vi "CoolProp_LogPH_SUBVI.vi"(9 "appended path":path, 10 "HoejTryk":dbl=-1111111111.0 format="%#.6f", 11 "Lavtryk":dbl=-1111111111.0 format="%#.6f") -> (0 "LogPH":cluster{dbl[], dbl[]}[](array[cluster]), 1 "Punkt4":T1, 2 "Punkt3":T1, 3 "Punkt1":T1, 5 "Punkt2":T1)   [LabVIEW 2022 SP3]
uses:
  Coolprop_64bit/CoolProp_advanced.llb/FluidCommon.ctl
  Coolprop_64bit/CoolProp_advanced.llb/FluidOfInterest.ctl
  Coolprop_64bit/Coolprop_lib.lvlib
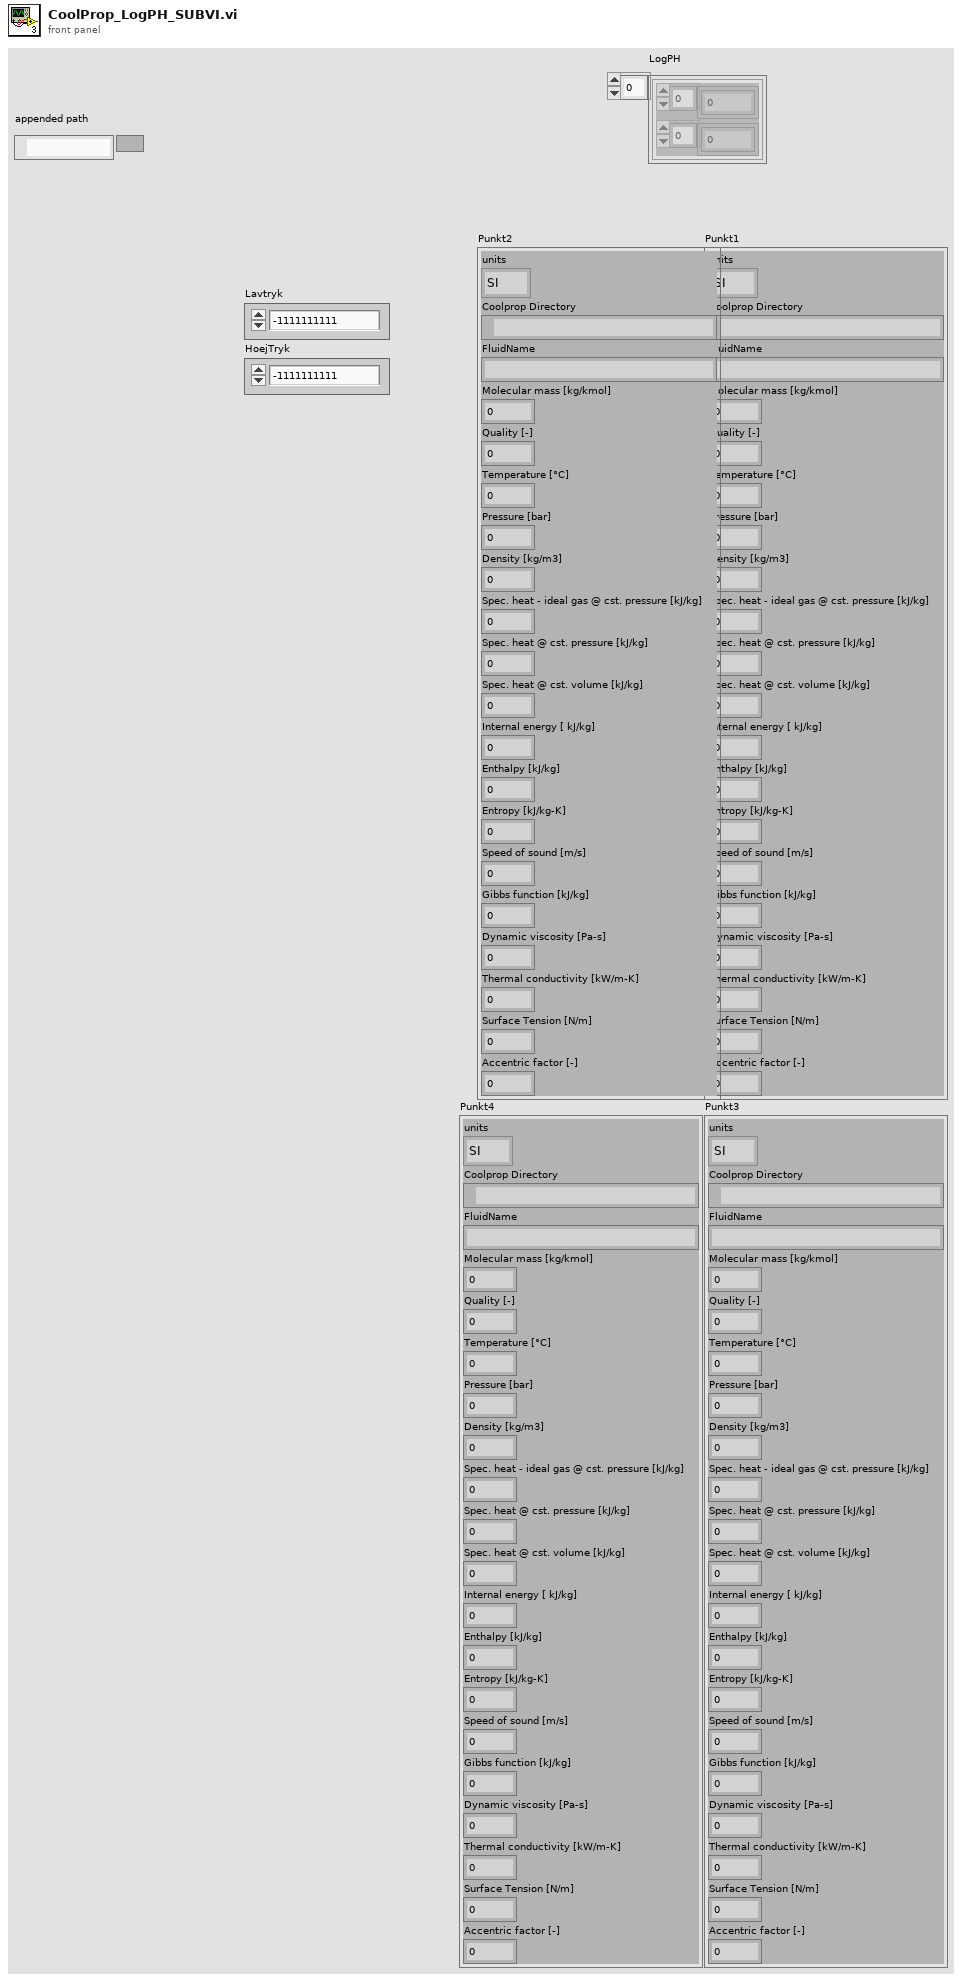
[diagram p1: front panel]
types:
  T1 = typedef "Coolprop_lib.lvlib/FluidCommon.ctl" = cluster{"units":enum16{"SI", "IP"}, "Coolprop Directory":path, "FluidName":string, "Molecular mass [kg/kmol]":dbl, "Quality [-]":dbl, "Temperature [°C]":dbl, "Pressure [bar]":dbl, "Density [kg/m3]":dbl, "Spec. heat - ideal gas @ cst. pressure [kJ/kg]":dbl, "Spec. heat @ cst. pressure [kJ/kg]":dbl, "Spec. heat @ cst. volume [kJ/kg]":dbl, "Internal energy [ kJ/kg]":dbl, "Enthalpy [kJ/kg]":dbl, "Entropy [kJ/kg-K]":dbl, "Speed of sound [m/s]":dbl, "Gibbs function [kJ/kg]":dbl, "Dynamic viscosity [Pa-s]":dbl, "Thermal conductivity [kW/m-K]":dbl, "Surface Tension [N/m]":dbl, "Accentric factor [-]":dbl}
  T2 = typedef "Coolprop_lib.lvlib/FluidOfInterest.ctl" = string
  T3 = enum16{"0", "TP", "TD", "PD", "TQ", "PQ", "HP", "SP", "SH"}
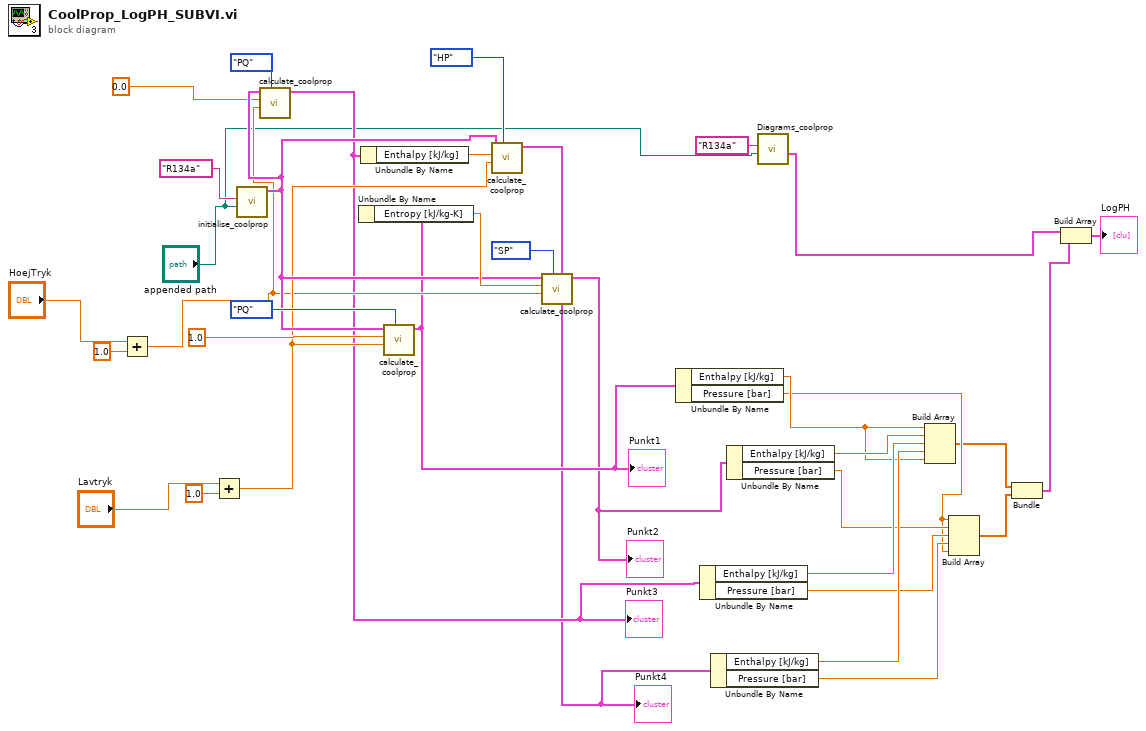
[diagram p0: block diagram]
diagram:
  n1 = Add(x="HoejTryk", y=1.0) -> (x+y=w20:dbl)
  n2 = Add(x="Lavtryk", y=1.0) -> (x+y=w23:dbl)
  n3 = call "initialise_coolprop.vi"("Path to CoolProp.dll"="appended path", "FluidOfInterest"=T2 "R134a") -> ("Common Out"=w28:T1)  [unwired: 7 in, 2 out]
  n4 = call "calculate_coolprop.vi"("InputCode"=T3."PQ", "Input_2"=w20, "Input_1"=0.0, "Common In"=w28) -> ("Common Out"=w17:T1)  [unwired: 3 in, 1 out]
  "Punkt3" <- w17
  n5 = Unbundle By Name(w17) -> ("Enthalpy [kJ/kg]"=w29:dbl)
  n6 = call "calculate_coolprop.vi"("InputCode"=T3."PQ", "Input_2"=w23, "Input_1"=1.0, "Common In"=w28) -> ("Common Out"=w19:T1)  [unwired: 3 in, 1 out]
  "Punkt1" <- w19
  n7 = Unbundle By Name(w19) -> ("Entropy [kJ/kg-K]"=w32:dbl)
  n8 = call "calculate_coolprop.vi"("InputCode"=T3."HP", "Input_2"=w23, "Input_1"=w29, "Common In"=w28) -> ("Common Out"=w16:T1)  [unwired: 3 in, 1 out]
  "Punkt4" <- w16
  n9 = call "calculate_coolprop.vi"("InputCode"=T3."SP", "Input_2"=w20, "Input_1"=w32, "Common In"=w28) -> ("Common Out"=w18:T1)  [unwired: 3 in, 1 out]
  "Punkt2" <- w18
  n10 = Unbundle By Name(w19) -> ("Enthalpy [kJ/kg]"=w12:dbl, "Pressure [bar]"=w8:dbl)
  n11 = Unbundle By Name(w17) -> ("Enthalpy [kJ/kg]"=w14:dbl, "Pressure [bar]"=w10:dbl)
  n12 = Unbundle By Name(w16) -> ("Enthalpy [kJ/kg]"=w13:dbl, "Pressure [bar]"=w9:dbl)
  n13 = Unbundle By Name(w18) -> ("Enthalpy [kJ/kg]"=w15:dbl, "Pressure [bar]"=w11:dbl)
  n14 = call "Diagrams_coolprop.vi"("Path"="appended path", "FluidOfInterest"=T2 "R134a") -> ("ph"=w2:cluster{dbl[], dbl[]})  [unwired: 2 in, 7 out]
  n15 = Build Array(w12, w15, w14, w13, w12) -> (w7:dbl[])
  n16 = Build Array(w8, w11, w10, w9, w8) -> (w6:dbl[])
  n17 = Bundle(w7, w6) -> (w3:cluster{dbl[], dbl[]})  [unwired: 1 in]
  n18 = Build Array(w2, w3) -> (→"LogPH":cluster{dbl[], dbl[]}[])
